vi "Task Type.vi"(8 "error in (no error)":errorcluster, 11 "Task in":refnum<class "Task.lvclass">) -> (0 "error out":errorcluster, 2 "Task Type":string, 3 "Task out":refnum<class "Task.lvclass">)   [LabVIEW 2020, in "VolatusConfig.lvlib" / "Task.lvclass"]
uses:
  Task.lvclass
  Task.lvclass/Task.ctl
  lv-cdm/CDM-Config/Config Element/Config Element.lvclass
  Meta Name.ctl
  VolatusConfig.lvlib
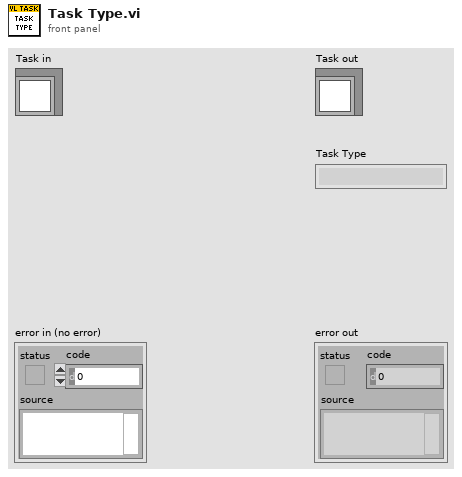
[diagram p1: front panel]
types:
  T1 = typedef "VolatusConfig.lvlib/Meta Name.ctl" = enum16{"VL_Type", "VL_Node_IP", "VL_Node_Type", "VL_Task_Type", "VL_Group_Type", "VL_Channel_Type", "VL_Channel_DataType"}
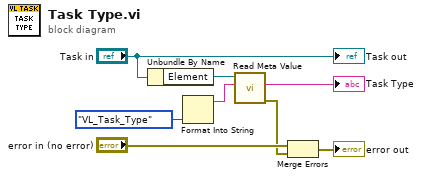
[diagram p0: block diagram]
diagram:
  n1 = Unbundle By Name("Task in") -> ("Element"=w6:refnum<class "Config Element.lvclass">)
  n2 = Format Into String(Meta_Name."VL_Task_Type" ("Meta Name")) -> (resulting string=w4:string)  [unwired: 3 in, 1 out]
  n3 = call "Read Meta Value.vi"("Meta Name"=w4, "Config Element in"=w6) -> ("error out"=w1:errorcluster, "Meta Value"=→"Task Type":string)  [unwired: 7 in, 1 out]
  n4 = Merge Errors("error in (no error)", w1) -> (→"error out":errorcluster)
  "Task out" <- "Task in"
